vi "Next step.vi"(8 "Auto cycle checks in":T2, 11 "Auto cycle step in":T1) -> (0 "Auto cycle checks out":T2, 3 "Auto cycle step out":T1)   [LabVIEW 2017, in "Auto cycle.lvlib"]
uses:
  Auto cycle.lvlib
  Controls/Checks.ctl
  Controls/Steps.ctl
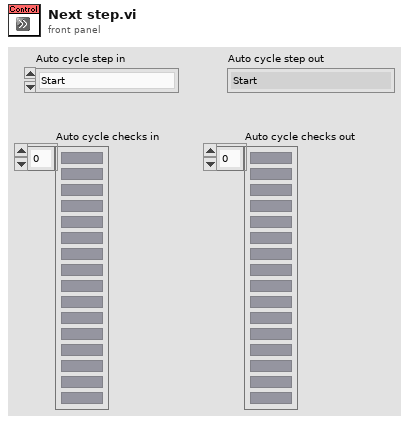
[diagram p1: front panel]
types:
  T1 = typedef "Auto cycle.lvlib/Steps.ctl" = enum16{"Start", "Setup spectrum", "Setup monochromator", "Setup colour wheel", "Move shutter", "Collect data", "Process A or B test", "A-B processing, stitching", "Return shutter"}
  T2 = typedef "Auto cycle.lvlib/Checks.ctl" = bool[]
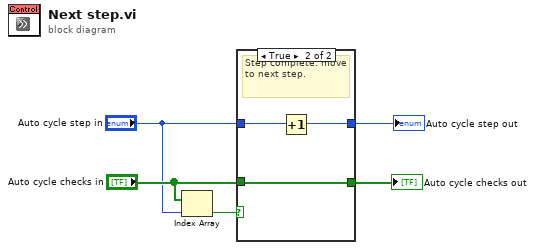
[diagram p0: block diagram]
diagram:
  n1 = Index Array(array="Auto cycle checks in", index="Auto cycle step in") -> (element=w3:bool)
  n2 = case shown="True" w3 {
    tunnel: [w6 w8] -> w2
    tunnel: "Auto cycle checks in" -> [w7 w10]
    tunnel: [w7 w10] -> w5
    tunnel: "Auto cycle step in" -> [w6 w9]
    frame False {
      # "Step requirements not met"
    }
    frame True {
      # "Step complete. move to next step."
      n3 = Increment(x=w9) -> (x+1=w8:T1)
    }
  }
  "Auto cycle checks out" <- w5
  "Auto cycle step out" <- w2
